vi "transport char run_subvi_2014_05_30_JWb.vi"(0 "VISA session":refnum<visa-resource-name>="GPIB0::17::INSTR", 1 "Y2 axis settings":T5={"Y2 axis on/off"=TRUE, "MINIMUM"=-1e-07, "MAXIMUM"=1e-07, "Variable name"="Ig", "LIN or LOG axis"=""} {"MAXIMUM" format="%.2e"; "MINIMUM" format="%.2e"}, 5 "Var1 sweep settings":T7={"start"=0.0, "stop"=-60.0, "step (linear only)"=-1.0, "sweep spacing (linear: 0)"=0, "sweep mode"=FALSE, "compliance (V)"=100.0, "compliance (A)"=0.001} {"compliance (A)" format="%^.2e"; "compliance (V)" format="%.2f"; "sweep spacing (linear: 0)" items=["linear", "log 10", "log 25", "log 50"]; "step (linear only)" format="%.2f"; "stop" format="%.2f"; "start" format="%.2f"}, 7 "Var2 step settings":T6={"compliance (A)"=0.001, "compliance (V)"=100.0, "start"=0.0, "total points"=7, "step"=-10.0} {"step" format="%.2f"; "start" format="%.2f"; "compliance (V)" format="%.2f"; "compliance (A)" format="%^.2e"}, 9 "integration time":u32(slide) scale=0.0..2.0, 11 "Path":path, 12 "SMU Config":T2={"Vname"="Vs", "Vname 2"="Vd", "Vname 3"="Vg", "Vname 4"="V4", "Iname"="Is", "Iname 2"="Id", "Iname 3"="Ig", "Iname 4"="I4", "Mode"=4, "Mode 2"=0, "Mode 3"=0, "Mode 4"=0, "Function"=4, "Function 2"=1, "Function 3"=2, "Function 4"=4, "Value (V or A)"=0.0, "Value (Either V or A) 2"=0.0, "Value (Either V or A) 3"=0.0, "Value (Either V or A) 4"=0.0} {"Function" items=["disabled", "Var1", "Var2", "Var1'", "Constant"]; "Mode" items=["V", "I", "VPulse", "IPulse", "Common"]; "Function 4" items=["disabled", "Var1", "Var2", "Var1'", "Constant"]; "Mode 4" items=["V", "I", "VPulse", "IPulse", "Common"]; "Function 3" items=["disabled", "Var1", "Var2", "Var1'", "Constant"]; "Mode 3" items=["V", "I", "VPulse", "IPulse", "Common"]; "Function 2" items=["disabled", "Var1", "Var2", "Var1'", "Constant"]; "Mode 2" items=["V", "I", "VPulse", "IPulse", "Common"]}, 13 "Sample Properties:":T4 {"Date Created" format="%<%Y/%m/%d>T"}, 14 "Ambient Temp (Y/N)":bool, 15 "error?":errorcluster) -> (6 "graphic display":cluster{"trace":dbl[], "trace":dbl[]}(graph), 8 "Graph Cluster":T3, 10 "Error Out":errorcluster)   [LabVIEW 2012]
uses:
  <vilib>/Utility/file.llb/Write To Spreadsheet File (DBL).vi
panel:
  in  "Y1 Axis Settings":T1={"Y1 axis"="Id", "MINIMUM"=-1e-05, "MAXIMUM"=0.0, "LIN or LOG axis"="LIN"} {"MAXIMUM" format="%.2e"; "MINIMUM" format="%_2e"}
  in  "Temp (K)":dbl=100.0 format="%^.2e"
  out "Gate Current Plot":cluster{"trace":dbl[], "trace":dbl[]}(graph)
  in  "wait time parameter":dbl=1.0
  in  "compliance (A)":dbl=0.001 format="%^.2e"
  in  "compliance (V)":dbl=100.0 format="%^.2e"
  in  "reset":bool=TRUE
  # "SMU1"
  # "SMU2"
  # "SMU3"
  # "SMU4"
  # "%"
  # "nm"
  # "Device Properties:"
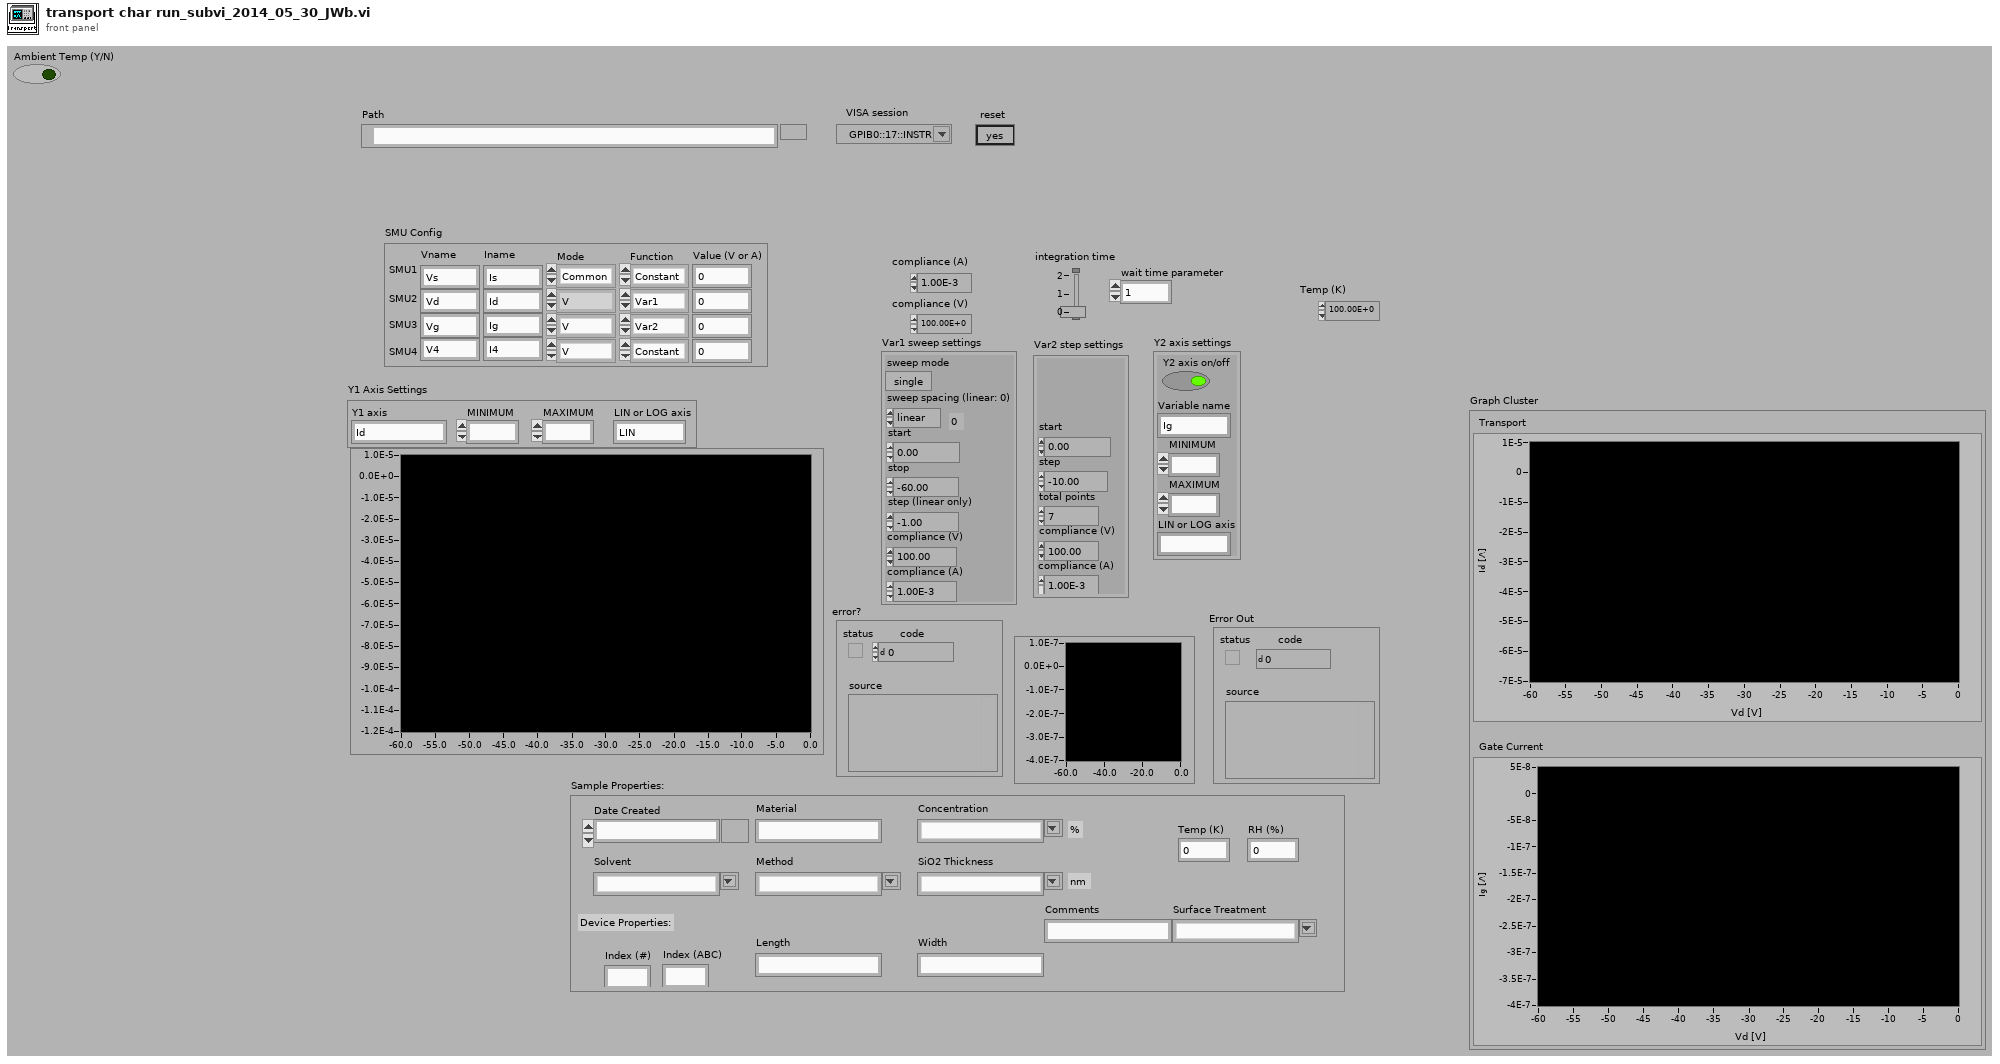
[diagram p1: front panel]
types:
  T1 = cluster{"Y1 axis":string, "MINIMUM":ext, "MAXIMUM":ext, "LIN or LOG axis":string}
  T2 = cluster{"Vname":string, "Vname 2":string, "Vname 3":string, "Vname 4":string, "Iname":string, "Iname 2":string, "Iname 3":string, "Iname 4":string, "Mode":u16, "Mode 2":u16, "Mode 3":u16, "Mode 4":u16, "Function":u16, "Function 2":u16, "Function 3":u16, "Function 4":u16, "Value (V or A)":dbl, "Value (Either V or A) 2":dbl, "Value (Either V or A) 3":dbl, "Value (Either V or A) 4":dbl}
  T3 = cluster{"Transport":cluster{dbl[], dbl[]}[], "Gate Current":cluster{dbl[], dbl[]}[]}
  T4 = cluster{"Date Created":timestamp, "Material":string, "Solvent":string, "Concentration":string, "Method":string, "SiO2 Thickness":string, "Index (#)":string, "Index (ABC)":string, "Length":string, "Width":string, "Surface Treatment":string, "Comments":string, "Temp (K)":dbl, "RH (%)":dbl}
  T5 = cluster{"Y2 axis on/off":bool, "MINIMUM":ext, "MAXIMUM":ext, "Variable name":string, "LIN or LOG axis":string}
  T6 = cluster{"compliance (A)":dbl, "compliance (V)":dbl, "start":dbl, "total points":u16, "step":dbl}
  T7 = cluster{"start":dbl, "stop":dbl, "step (linear only)":dbl, "sweep spacing (linear: 0)":u16, "sweep mode":bool, "compliance (V)":dbl, "compliance (A)":dbl}
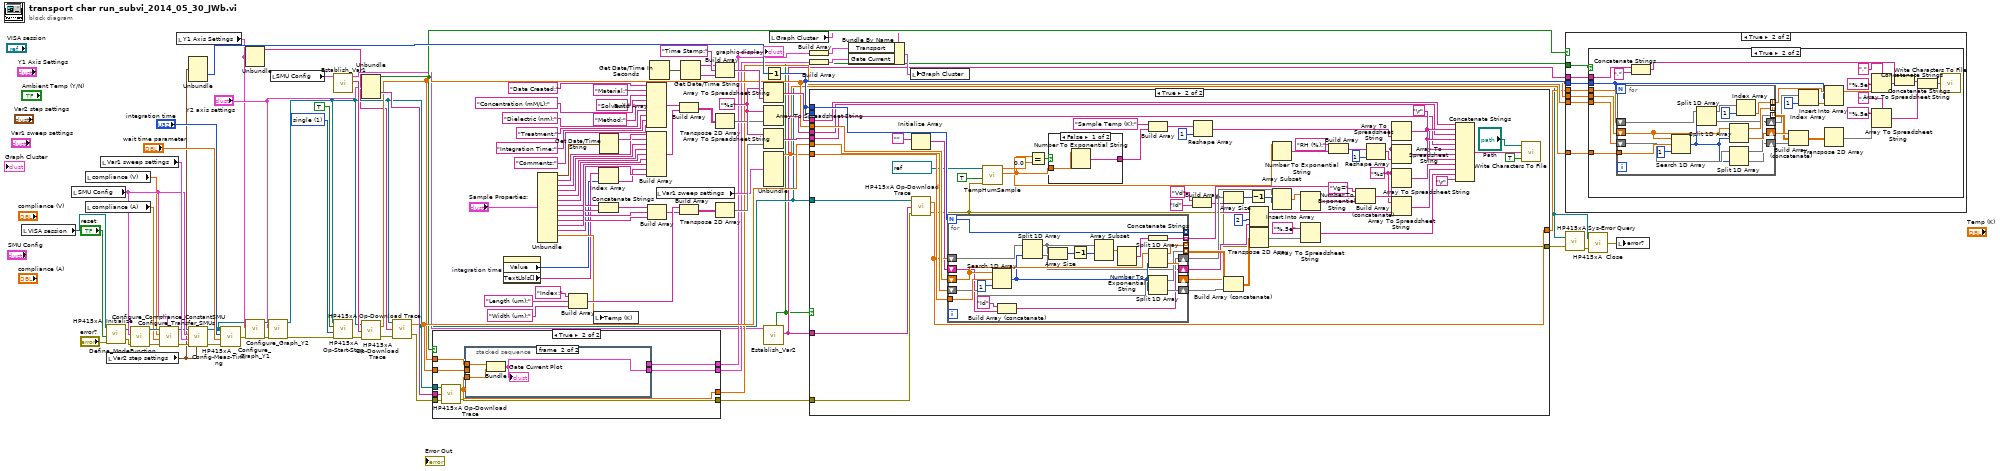
[diagram p0: block diagram]
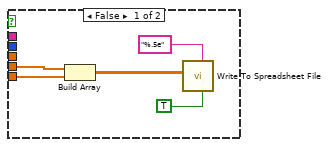
[diagram p3: hidden frame]
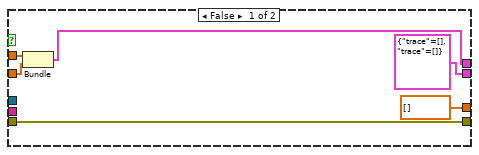
[diagram p4: hidden frame]
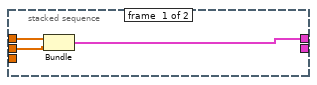
[diagram p5: hidden frame]
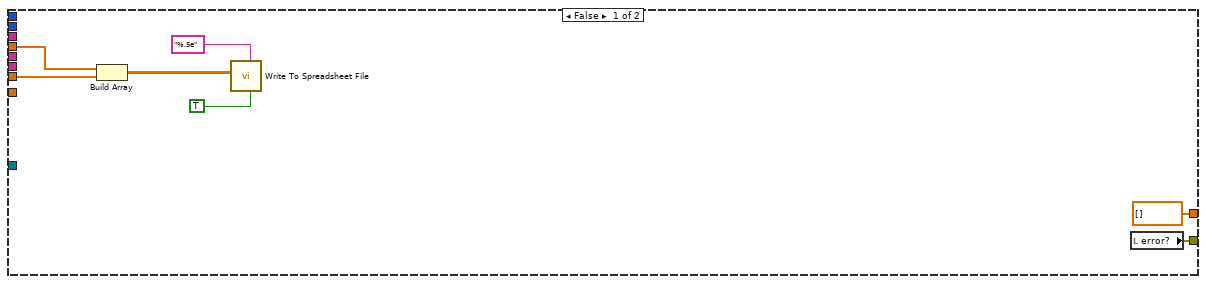
[diagram p6: hidden frame]
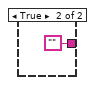
[diagram p7: hidden frame]
diagram:
  w35 = u32 1 items=["stop  ", "single  ", "single-append  ", "stress start  ", "continuous  ", "standby on  ", "standby off  ", "zero  "] ("function (stop:0)")
  w92 = "%s"
  n1 = local read "VISA session"() -> (w3:refnum<visa-resource-name>)
  n2 = local read "SMU Config"() -> (w51:T2)
  n3 = local read "compliance (V)"() -> (w46:dbl)
  n4 = local read "compliance (A)"() -> (w47:dbl)
  n5 = local read "Var1 sweep settings"() -> (w52:T7)
  n6 = call "HP415xA  Initialize.vi"("instrument descriptor"=w3, "reset"="reset", "error in (no error)"="error?") -> ("VISA session"=w44:refnum<visa-resource-name>, "error out"=w45:errorcluster)  [unwired: 2 in]
  n7 = local read "Var2 step settings"() -> (w1:T6)
  n8 = call "Define_ModeFunction.vi"("error in (no error)"=w45, "SMU Config"=w51, "VISA Refnum in"=w44) -> ("error out"=w48:errorcluster, "VISA Refnum out"=w49:refnum<visa-resource-name>)  [unwired: 7 in]
  n9 = call "Configure_Compliance_ConstantSMU.vi"("SMU Config"=w51, "error in (no error)"=w48, "compliance (A)"=w47, "compliance (V)"=w46, "VISA In"=w49) -> ("error out"=w53:errorcluster, "VISA Out"=w50:refnum<visa-resource-name>)  [unwired: 5 in]
  n10 = local read "Y1 Axis Settings"() -> (w8:T1)
  n11 = Unbundle(w1) -> ("total points"=w37:u16)  [unwired: 4 out]
  n12 = call "Configure_Transfer_SMUs.vi"("Var2 step settings"=w1, "error in (no error)"=w53, "Var1 sweep settings"=w52, "SMU Config"=w51, "VISA In"=w50) -> ("error out"=w56:errorcluster, "VISA Out"=w2:refnum<visa-resource-name>)  [unwired: 5 in]
  n13 = call "HP415xA _Config-Meas-Timing.vi"("error in (no error)"=w56, "wait time parameter"="wait time parameter", "integration time"="integration time", "VISA session"=w2) -> ("error out"=w4:errorcluster)  [unwired: 2 in]
  n14 = Unbundle(w8) -> ("Y1 axis"=w7:string)  [unwired: 3 out]
  n15 = call "Configure_Graph_Y1.vi"("error in (no error)"=w4, "Y1 Axis Settings"=w8, "VISA In"=w2) -> ("error out"=w10:errorcluster, "VISA Out"=w13:refnum<visa-resource-name>)  [unwired: 7 in]
  n16 = call "Configure_Graph_Y2.vi"("error in (no error)"=w10, "Y2 axis settings"="Y2 axis settings", "VISA In"=w13) -> ("error out"=w11:errorcluster, "VISA Out"=w9:refnum<visa-resource-name>)  [unwired: 7 in]
  n17 = local read "SMU Config"() -> (w16:T2)
  n18 = call "Establish_Var1.vi"("SMU Config In"=w16) -> ("Vname"=w14:string, "SMU Config Out"=w15:T2)  [unwired: 8 in]
  n19 = call "HP415xA Op-Start-Stop.vi"("error in (no error)"=w11, "function (stop:0)"=w35, "wait until finish"=TRUE, "VISA session"=w9) -> ("error out"=w34:errorcluster)  [unwired: 6 in, 1 out]
  n20 = Unbundle("Y2 axis settings") -> ("Y2 axis on/off"=w29:bool, "Variable name"=w32:string)  [unwired: 3 out]
  n21 = call "HP415xA Op-Download Trace.vi"("error in (no error)"=w34, "trace (variable) name"=w14, "VISA session"=w9) -> ("error out"=w41:errorcluster, "trace"=w27:dbl[])
  n22 = call "HP415xA Op-Download Trace.vi"("error in (no error)"=w41, "trace (variable) name"=w7, "VISA session"=w9) -> ("error out"=w33:errorcluster, "trace"=w30:dbl[])
  n23 = case shown="True" w29 {
    tunnel: w33 -> [w110 w119]
    tunnel: w9 -> [_ w118]
    tunnel: w32 -> [_ w117]
    tunnel: [w110 w116] -> w31
    tunnel: w27 -> [w108 w115]
    tunnel: w30 -> [w109 w114]
    tunnel: [w107 w113] -> w19
    tunnel: [dbl[] [] ("trace") w112] -> w25
    tunnel: [cluster{"trace":dbl[], "trace":dbl[]} {"trace"=[], "trace"=[]} w111] -> w17
    frame False {
      n24 = Bundle("trace"=w108, "trace"=w109) -> (w107:cluster{"trace":dbl[], "trace":dbl[]})  [unwired: 1 in]
    }
    frame True {
      n25 = call "HP415xA Op-Download Trace.vi"("error in (no error)"=w119, "trace (variable) name"=w117, "VISA session"=w118) -> ("error out"=w116:errorcluster, "trace"=w112:dbl[])
      n26 = stacked-sequence {
        tunnel: w112 -> [_ w125]
        tunnel: w115 -> [w122 w124]
        tunnel: w114 -> [w121 _]
        tunnel: [w120 _] -> w113
        tunnel: [_ w123] -> w111
        frame #0 {
          n27 = Bundle("trace"=w122, "trace"=w121) -> (w120:cluster{"trace":dbl[], "trace":dbl[]})  [unwired: 1 in]
        }
        frame #1 {
          n28 = Bundle("trace"=w124, "trace"=w125) -> (w123:cluster{"trace":dbl[], "trace":dbl[]})  [unwired: 1 in]
          "Gate Current Plot" <- w123
        }
      }
    }
  }
  "graphic display" <- w19
  n29 = property on="integration time" class="Slide (strict)"() -> ("Value"=w60:u32, "TextLbls[]"=w61:string[])  [unwired: 2 in, 2 out]
  n30 = Unbundle("Sample Properties:") -> ("Date Created"=w76:timestamp, "Material"=w75:string, "Solvent"=w72:string, "Concentration"=w70:string, "Method"=w74:string, "SiO2 Thickness"=w71:string, "Index (#)"=w68:string, "Index (ABC)"=w67:string, "Length"=w65:string, "Width"=w64:string, "Surface Treatment"=w69:string, "Comments"=w59:string, "Temp (K)"=w63:dbl)  [unwired: 1 out]
  n31 = Build Array("Index:", "Length (um):", "Width (um):") -> (w81:string[])
  n32 = local write "Temp (K)"(w63) -> ()
  n33 = Index Array(array=w61, index=w60) -> (element=w58:string)
  n34 = Concatenate Strings(w68, w67) -> (w66:string)
  n35 = Get Date/Time String(seconds (now)=w76) -> (date string=w104:string)  [unwired: 2 in, 1 out]
  n36 = Build Array("Date Created:", "Material:", "Solvent:", "Concentration (mM/L):", "Method:", "Dielectric (nm):", "Treatment:", "Integration Time:", "Comments:") -> (w85:string[])
  n37 = Build Array(w104, w75, w72, w70, w74, w71, w69, w58, w59) -> (w84:string[])
  n38 = Build Array(w66, w65, w64) -> (w80:string[])
  n39 = Get Date/Time In Seconds() -> (seconds since 1Jan1904=w99:timestamp)
  n40 = local read "Var1 sweep settings"() -> (w38:T7)
  n41 = Build Array(w85, w84) -> (w83:string[][])
  n42 = Build Array(w81, w80) -> (w79:string[][])
  n43 = Get Date/Time String(seconds (now)=w99) -> (date string=w98:string, time string=w97:string)  [unwired: 2 in]
  n44 = Build Array("Time Stamp:", w98, w97) -> (w96:string[])
  n45 = Transpose 2D Array(2D array=w83) -> (transposed array=w82:string[][])
  n46 = Transpose 2D Array(2D array=w79) -> (transposed array=w78:string[][])
  n47 = Array To Spreadsheet String(array=w96, 3:w92) -> (spreadsheet string=w91:string)  [unwired: 1 in]
  n48 = Array To Spreadsheet String(array=w82, 3:w92) -> (spreadsheet string=w90:string)  [unwired: 1 in]
  n49 = Array To Spreadsheet String(array=w78, 3:w92) -> (spreadsheet string=w89:string)  [unwired: 1 in]
  n50 = Unbundle(w38) -> ("start"=w26:dbl)  [unwired: 6 out]
  n51 = call "Establish_Var2.vi"("SMU Config In"=w15) -> ("Vname"=w6:string, "Execute?"=w5:bool)  [unwired: 8 in, 1 out]
  n52 = Decrement(x=w37) -> (x-1=w28:u16)
  n53 = local read "Graph Cluster"() -> (w22:T3)
  n54 = Build Array(w19) -> (w20:cluster{"trace":dbl[], "trace":dbl[]}[])
  n55 = Build Array(w17) -> (w18:cluster{"trace":dbl[], "trace":dbl[]}[])
  n56 = case shown="True" w5 {
    tunnel: w26 -> [_ w193]
    tunnel: w30 -> [w130 w192]
    tunnel: w27 -> [w131 w190]
    tunnel: w28 -> [_ w188]
    tunnel: w28 -> [_ _]
    tunnel: w9 -> [_ w184]
    tunnel: w31 -> [_ w183]
    tunnel: [w132 w138] -> w23
    tunnel: [dbl[] [] ("trace") w182] -> w24
    tunnel: w91 -> [_ w177]
    tunnel: w90 -> [_ w176]
    tunnel: w89 -> [_ w175]
    tunnel: w6 -> [_ w133]
    frame False {
      n57 = Build Array(w131, w130) -> (w127:dbl[][])
      n58 = call-poly <vilib>:"Write To Spreadsheet File.vi"("transpose? (no:F)"=TRUE ("append to file? (new file:F)"), "format (%.3f)"="%.5e", "2D data"=w127) -> ()  [unwired: 5 in, 1 out]
      n59 = local read "error?"() -> (w132:errorcluster)
    }
    frame True {
      w140 = "%s"
      w179 = "\r"
      n60 = Initialize Array("") -> (w157:string[])  [unwired: 1 in]
      n61 = call "HP415xA Op-Download Trace.vi"("error in (no error)"=w183, "trace (variable) name"=w133, "VISA session"=w184) -> ("error out"=w138:errorcluster, "trace"=w182:dbl[])
      n62 = for {
        N: w188 -> [w197]
        shift-right: [w214] -> w163
        shift-left: w190 -> [w210]
        tunnel: w193 -> [w216]
        tunnel: [w215] -> _ mode=indexing
        shift-right: [w211] -> w189
        shift-left: w192 -> [w213]
        tunnel: [w212] -> w191 mode=indexing
        shift-right: [w207] -> w170
        shift-left: w182 -> [w209]
        tunnel: [w201] -> w172 mode=indexing
        shift-right: [w200] -> w161
        shift-left: w157 -> [w199]
        tunnel: [w197] -> _ mode=indexing
        n63 = Search 1D Array(1D array=w210, element=w216, start index (0)=1) -> (index of element=w208:i32)
        n64 = Build Array (concatenate)("Id", w199) -> (w200:string[])
        n65 = Split 1D Array(array=w209, index=w208) -> (first subarray=w205:dbl[], second subarray=w207:dbl[])
        n66 = Array Size(array=w205) -> (size(s)=w204:i32)
        n67 = Decrement(x=w204) -> (x-1=w203:i32)
        n68 = Array Subset(array=w205, index=w203) -> (w206:dbl[])  [unwired: 1 in]
        n69 = Number To Exponential String(number=w206) -> (E-format string=w202:string[])  [unwired: 3 in]
        n70 = Concatenate Strings(w202) -> (w201:string)
        n71 = Split 1D Array(array=w210, index=w208) -> (first subarray=w215:dbl[], second subarray=w214:dbl[])
        n72 = Split 1D Array(array=w213, index=w208) -> (first subarray=w212:dbl[], second subarray=w211:dbl[])
      }
      n73 = call "TempHumSample.vi"("VISA resource name"=refnum<visa-resource-name> "COM4", "Single Sample?"=TRUE, "error in (no error)"=w138) -> ("CurHum"=w134:dbl, "CurTemp"=w135:dbl)  [unwired: 5 in, 1 out]
      n74 = Equal?(x=w135, y=0.0) -> (x = y?=w148:bool)
      n75 = case shown="False" w148 {
        tunnel: w135 -> [w195 _]
        tunnel: [w194 ""] -> w146
        frame False {
          n76 = Number To Exponential String(number=w195) -> (E-format string=w194:string)  [unwired: 3 in]
        }
        frame True {
        }
      }
      n77 = Build Array("Sample Temp (K):", w146) -> (w152:string[])
      n78 = Build Array("Vd", "Id") -> (w162:string[])
      n79 = Reshape Array(w152, 1 ("start index (0)")) -> (w150:string[])
      n80 = Array Size(array=w170) -> (size(s)=w171:i32)
      n81 = Build Array (concatenate)(w163, w191, w189) -> (w187:dbl[][])
      n82 = Decrement(x=w171) -> (x-1=w169:i32)
      n83 = Insert Into Array(array=w162, index=2, new element=w161) -> (w160:string[])
      n84 = Transpose 2D Array(2D array=w187) -> (transposed array=w185:dbl[][])
      n85 = Number To Exponential String(number=w134) -> (E-format string=w142:string)  [unwired: 3 in]
      n86 = Array Subset(array=w170, index=w169) -> (w168:dbl[])  [unwired: 1 in]
      n87 = Number To Exponential String(number=w168) -> (E-format string=w154:string[])  [unwired: 3 in]
      n88 = Array To Spreadsheet String(array=w185, 3:"%.5e" ("format string")) -> (spreadsheet string=w174:string)  [unwired: 1 in]
      n89 = Build Array("RH (%):", w142) -> (w144:string[])
      n90 = Build Array (concatenate)("Vg=", w172, w154) -> (w167:string[])
      n91 = Reshape Array(w144, 1 ("start index (0)")) -> (w141:string[])
      n92 = Array To Spreadsheet String(array=w150, 3:w140) -> (spreadsheet string=w149:string)  [unwired: 1 in]
      n93 = Array To Spreadsheet String(array=w141, 3:w140) -> (spreadsheet string=w139:string)  [unwired: 1 in]
      n94 = Array To Spreadsheet String(array=w167, 3:w140) -> (spreadsheet string=w173:string)  [unwired: 1 in]
      n95 = Array To Spreadsheet String(array=w160, 3:w140) -> (spreadsheet string=w166:string)  [unwired: 1 in]
      n96 = Concatenate Strings(w177, w179, w176, w179, w175, w149, w139, w179, w173, w166, w174, "\r") -> (w181:string)
      n97 = call <vilib>:"Write Characters To File.vi"("append to file? (new file:F)"=TRUE, "character string"=w181, "file path (dialog if empty)"="Path") -> ()  [unwired: 2 in, 1 out]
    }
  }
  n98 = Bundle By Name(cluster=w22, "Transport"=w20, "Gate Current"=w18) -> (w21:T3)
  n99 = local write "Graph Cluster"(w21) -> ()
  n100 = case shown="True" w29 {
    tunnel: w28 -> [_ w224]
    tunnel: w27 -> [_ w223]
    tunnel: w26 -> [_ w222]
    tunnel: w25 -> [_ w221]
    tunnel: w24 -> [_ w220]
    tunnel: w6 -> [_ w219]
    tunnel: w5 -> [_ w218]
    frame False {
    }
    frame True {
      n101 = case shown="True" w218 {
        tunnel: w224 -> [_ w240]
        tunnel: w223 -> [w228 w255]
        tunnel: w222 -> [_ w254]
        tunnel: w221 -> [w229 w253]
        tunnel: w220 -> [_ w252]
        tunnel: w219 -> [_ w230]
        frame False {
          n102 = Build Array(w228, w229) -> (w227:dbl[][])
          n103 = call-poly <vilib>:"Write To Spreadsheet File.vi"("transpose? (no:F)"=TRUE, "format (%.3f)"="%.5e", "2D data"=w227) -> ()  [unwired: 5 in, 1 out]
        }
        frame True {
          n104 = for {
            N: w240 -> [_]
            shift-right: [w266] -> w251
            shift-left: w255 -> [w267]
            tunnel: w254 -> [w269]
            tunnel: [w265] -> _ mode=indexing
            shift-right: [w262] -> w249
            shift-left: w253 -> [w264]
            tunnel: [w263] -> w250 mode=indexing
            shift-right: [w259] -> w244
            shift-left: w252 -> [w260]
            tunnel: [w256] -> w241 mode=indexing
            n105 = Search 1D Array(1D array=w267, element=w269, start index (0)=1) -> (index of element=w261:i32)
            n106 = Split 1D Array(array=w260, index=w261) -> (first subarray=w257:dbl[], second subarray=w259:dbl[])
            n107 = Split 1D Array(array=w267, index=w261) -> (first subarray=w265:dbl[], second subarray=w266:dbl[])
            n108 = Split 1D Array(array=w264, index=w261) -> (first subarray=w263:dbl[], second subarray=w262:dbl[])
            n109 = Index Array(array=w257, index=1) -> (element=w256:dbl)
          }
          n110 = Concatenate Strings(w230, "," ("string")) -> (w235:string)
          n111 = Build Array (concatenate)(w251, w250, w249) -> (w248:dbl[][])
          n112 = Index Array(array=w244, index=1) -> (element=w242:dbl)
          n113 = Insert Into Array(array=w241, index=w240, new element=w242) -> (w239:dbl[])
          n114 = Transpose 2D Array(2D array=w248) -> (transposed array=w247:dbl[][])
          n115 = Array To Spreadsheet String(delimiter (Tab)=",", array=w239, 3:"%.5e" ("format string")) -> (spreadsheet string=w234:string)
          n116 = Array To Spreadsheet String(delimiter (Tab)=",", array=w247, 3:"%.5e" ("format string")) -> (spreadsheet string=w232:string)
          n117 = Concatenate Strings(w235, w234) -> (w233:string)
          n118 = Concatenate Strings(w233, w232) -> (w231:string)
          n119 = call <vilib>:"Write Characters To File.vi"("character string"=w231) -> ()  [unwired: 4 in, 1 out]
        }
      }
    }
  }
  n120 = call "HP415xA Sys-Error Query.vi"("VISA session"=w9, "error in (no error)"=w23) -> ("error out"=w39:errorcluster)  [unwired: 2 in, 1 out]
  n121 = call "HP415xA  Close.vi"("error in (no error)"=w39, "VISA session"=w9) -> ("error out"=w40:errorcluster)
  n122 = local write "error?"(w40) -> ()
